vi "RGBtoColor.vi"(1 "RGB":dbl[](array[numeric])) -> (0 "Color":u32(colorbox))   [LabVIEW 2013]
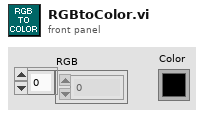
[diagram p1: front panel]
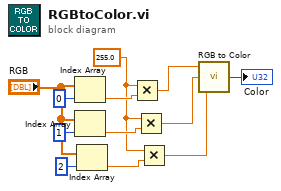
[diagram p0: block diagram]
diagram:
  w6 = 255.0
  n1 = Index Array(array="RGB", index=0) -> (element=w9:dbl)
  n2 = Index Array(array="RGB", index=1) -> (element=w7:dbl)
  n3 = Index Array(array="RGB", index=2) -> (element=w8:dbl)
  n4 = Multiply(x=w6, y=w9) -> (x*y=w5:dbl)
  n5 = Multiply(x=w6, y=w7) -> (x*y=w4:dbl)
  n6 = Multiply(x=w6, y=w8) -> (x*y=w3:dbl)
  n7 = call <vilib>:"RGB to Color.vi"("B"=w3, "G"=w4, "R"=w5) -> ("Color"=→"Color":u32)
